vi "SDCP - Get Frame IDs.vi"(2 "error in (no error)":errorcluster, 3 "Frame names":string[](array[string])) -> (0 "error out":errorcluster, 1 "Frame IDs":u8[](array[numeric]))   [LabVIEW 2020]
uses:
  Typedefs/SDCP - Standard Message Frame Parameters - FGV - commands.ctl
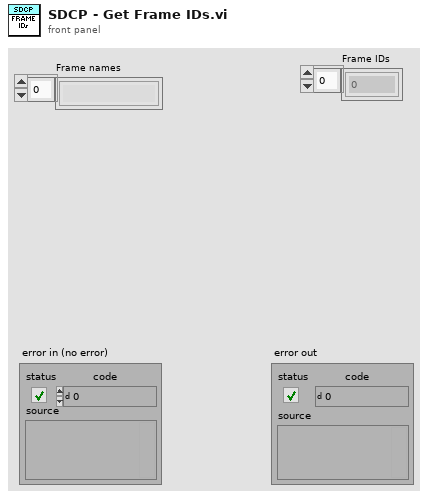
[diagram p1: front panel]
types:
  T1 = typedef "SDCP - Standard Message Frame Parameters - FGV - commands.ctl" = enum16{"Write descriptors", "Read descriptors", "Read values", "Load parameters from file", "Write values", "Read all descriptors"}
  T2 = typedef "SDCP - SMF parameter descriptors.ctl" = cluster{"Frame name":string, "Frame ID":i32, "Data type":string, "Start Position":i32, "Length":i32, "Factor":dbl, "Offset":dbl, "Parameter name":string, "Value":string}
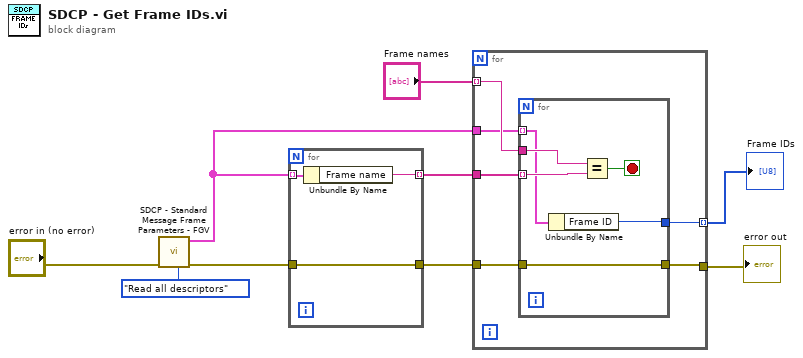
[diagram p0: block diagram]
diagram:
  n1 = call "SDCP - Standard Message Frame Parameters - FGV.vi"("error in (no error)"="error in (no error)", "Command"=SDCP_-_Standard_Message_Frame_Parameters_-_FGV_-_commands."Read all descriptors") -> ("SMF Parameters descriptors out"=w3:T2[], "error out"=w7:errorcluster)  [unwired: 5 in]
  n2 = for {
    tunnel: w7 -> [w10]
    tunnel: w3 -> [w12] mode=indexing
    tunnel: [w11] -> w4 mode=indexing
    tunnel: [w10] -> w5
    n3 = Unbundle By Name(w12) -> ("Frame name"=w11:string)
  }
  n4 = for {
    tunnel: "Frame names" -> [w16] mode=indexing
    tunnel: w5 -> [w18]
    tunnel: w4 -> [w17]
    tunnel: w3 -> [w15]
    tunnel: [w14] -> w1 mode=indexing
    tunnel: [w13] -> w2
    n5 = for {
      tunnel: w18 -> [w19]
      tunnel: w17 -> [w24] mode=indexing
      tunnel: w16 -> [w23]
      tunnel: w15 -> [w21] mode=indexing
      tunnel: [w20] -> w14
      tunnel: [w19] -> w13
      stop <- w22 stop-if-true
      n6 = Unbundle By Name(w21) -> ("Frame ID"=w20:i32)
      n7 = Equal?(x=w23, y=w24) -> (x = y?=w22:bool)
    }
  }
  "Frame IDs" <- w1
  "error out" <- w2
